vi "ex3.vi"() -> ()   [LabVIEW 2022 SP3]
panel:
  out "Weeks":dbl
  out "Minutues":dbl
  out "Seconds":dbl
  out "Hours":dbl
  out "Rest from the Hours":dbl
  out "Rest from the Days":dbl
  out "Rest from the Weeks":dbl
  out "Days":dbl
  in  "Seconds":dbl format="%#_10f"
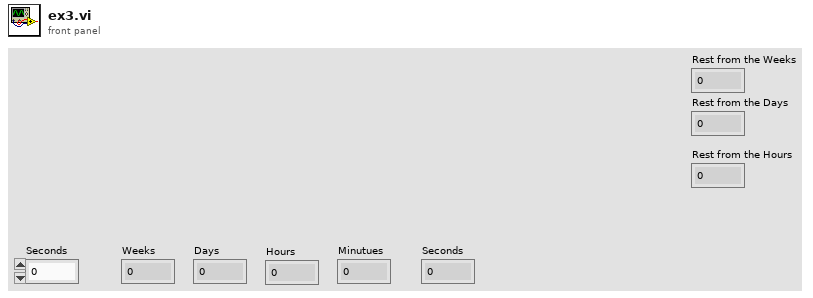
[diagram p1: front panel]
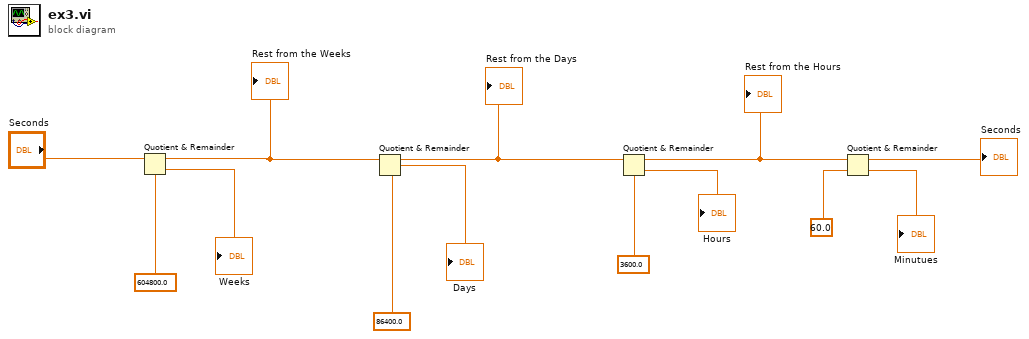
[diagram p0: block diagram]
diagram:
  n1 = Quotient & Remainder(x="Seconds", y=604800.0) -> (x-y*floor(x/y)=w11:dbl, floor(x/y)=→"Weeks":dbl)
  "Rest from the Weeks" <- w11
  n2 = Quotient & Remainder(x=w11, y=86400.0) -> (x-y*floor(x/y)=w8:dbl, floor(x/y)=→"Days":dbl)
  "Rest from the Days" <- w8
  n3 = Quotient & Remainder(x=w8, y=3600.0) -> (x-y*floor(x/y)=w5:dbl, floor(x/y)=→"Hours":dbl)
  "Rest from the Hours" <- w5
  n4 = Quotient & Remainder(x=w5, y=60.0) -> (x-y*floor(x/y)=→"Seconds":dbl, floor(x/y)=→"Minutues":dbl)
